vi "Get Reference to Single Transient Capture.vi"() -> (3 "VI out":refnum<vi>)   [LabVIEW 2017, in "DTACQ - Network Enabled Device Driver.lvlib"]
uses:
  DTACQ - Network Enabled Device Driver.lvlib
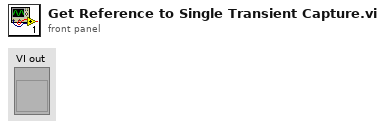
[diagram p1: front panel]
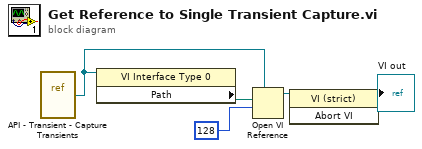
[diagram p0: block diagram]
diagram:
  n1 = vi-ref "API - Transient - Capture Transients.vi"() -> (w3:refnum<vi>)
  n2 = property class="VI Interface Type 0"(reference=w3) -> ("Path"=w2:path)  [unwired: 1 in, 2 out]
  n3 = Open VI Reference(type specifier VI Refnum (for type only)=w3, vi path=w2, options=128) -> (vi reference=w5:refnum<vi>)  [unwired: 3 in, 1 out]
  n4 = invoke class="VI (strict)" method="Abort VI"(reference=w5) -> (reference out=→"VI out":refnum<vi>)  [unwired: 2 in, 2 out]
